vi "To String.vi"(6 "Encoding [No encoding]":refnum<class "CConfig Encoding.lvclass">, 7 "Persitant only?":bool, 8 "error in (no error)":errorcluster, 9 "Prev. Newline":string, 11 "Section Object in":refnum<class "CConfig Object.lvclass">) -> (0 "error out":errorcluster, 1 "Next Newline":string, 2 "String":string, 3 "Section Object out":refnum<class "CConfig Object.lvclass">)   [LabVIEW 2013, in "CConfig Object.lvclass"]
doc: "Copyright 2018, Carya Automatisering, Wiebe Walstra."
uses:
  CConfig Object.lvclass
  CConfig Encoding/CConfig Encoding.lvclass
  CConfig Object.lvclass/CConfig Object.ctl
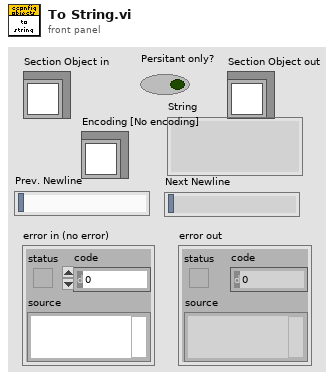
[diagram p1: front panel]
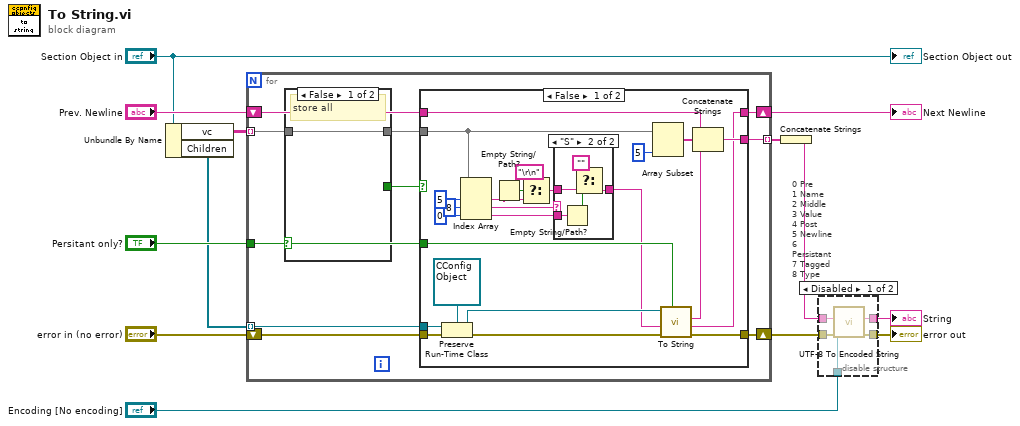
[diagram p0: block diagram]
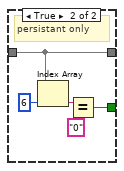
[diagram p3: hidden frame]
diagram:
  # "0 Pre\n1 Name\n2 Middle\n3 Value\n4 Post\n5 Newline\n6 Persistant\n7 Tagged\n8 Type"
  n1 = Unbundle By Name("Section Object in") -> ("vc"=w10:string[][], "Children"=w9:refnum<class>[])
  n2 = for {
    tunnel: [w23] -> w8 mode=indexing
    shift-right: [w22] -> w11
    shift-left: "error in (no error)" -> [w17]
    tunnel: "Persitant only?" -> [w15]
    tunnel: w10 -> [w19] mode=indexing
    tunnel: w9 -> [w18] mode=indexing
    shift-right: [w20] -> w4
    shift-left: "Prev. Newline" -> [w21]
    n3 = case shown="False" w15 {
      tunnel: w19 -> [w24 w25]
      tunnel: [_ w26] -> w16
      tunnel: [w24 w25] -> w14
      frame False {
        # "store all"
      }
      frame True {
        # "persistant only"
        n4 = Index Array(array=w25, index=6) -> (element=w27:string)
        n5 = Equal?(x=w27, y="0") -> (x = y?=w26:bool)
      }
    }
    n6 = case shown="False" w16 {
      tunnel: [w53 _] -> w23
      tunnel: w15 -> [w52 _]
      tunnel: [w51 w61] -> w22
      tunnel: w21 -> [w47 w60]
      tunnel: [w46 w60] -> w20
      tunnel: w14 -> [w40 _]
      tunnel: w17 -> [w45 w61]
      tunnel: w18 -> [w41 _]
      frame False {
        n7 = Preserve Run-Time Class(object in=w41, error in=w45, 2:refnum<class "CConfig Object.lvclass"> refnum ("Composite Object.lvclass")) -> (object out=w43:refnum<class "CConfig Object.lvclass">, error out=w44:errorcluster)
        n8 = Index Array(array=w40, index #1=5 ("index"), index #2=8 ("index"), index #3=0 ("index")) -> (element #1=w39:string, element #2=w33:string, element #3=w30:string)
        n9 = Empty String/Path?(string/path=w39) -> (empty?=w35:bool)
        n10 = Select(t="\r\n", s=w35, f=w39) -> (s? t:f=w32:string)
        n11 = case shown="\"S\"" w33 {
          tunnel: [w54 w56] -> w31
          tunnel: w32 -> [w54 w57]
          tunnel: w30 -> [_ w59]
          frame Default {
          }
          frame "S" {
            n12 = Empty String/Path?(string/path=w59) -> (empty?=w58:bool)
            n13 = Select(t="", s=w58, f=w57) -> (s? t:f=w56:string)
          }
        }
        n14 = Array Subset(array=w40, length=5 ("index")) -> (w49:string[])  [unwired: 1 in]
        n15 = call-dynamic "To String.vi"("Persitant only?"=w52, "error in (no error)"=w44, "Prev. Newline"=w31, "Section Object in"=w43) -> ("error out"=w51:errorcluster, "Next Newline"=w46:string, "String"=w50:string)  [unwired: 4 in, 1 out]
        n16 = Concatenate Strings(w47, w49, w50) -> (w53:string)
      }
      frame True {
      }
    }
  }
  "Next Newline" <- w4
  n17 = Concatenate Strings(w8) -> (w2:string)
  n18 = disable-structure shown="Disabled" {
    disable-tunnel: w11 -> [w66 w67]
    disable-tunnel: [w65 w67] -> w6
    disable-tunnel: [w64 w68] -> w3
    disable-tunnel: w2 -> [w63 w68]
    disable-tunnel: "Encoding [No encoding]" -> [w62 _]
    frame Disabled {
      n19 = call-dynamic "UTF-8 To Encoded String.vi"("error in (no error)"=w66, "UTF-8 string"=w63, "Encoding in"=w62) -> ("error out"=w65:errorcluster, "Encoded string"=w64:string)  [unwired: 6 in, 1 out]
    }
    frame Enabled {
    }
  }
  "error out" <- w6
  "String" <- w3
  "Section Object out" <- "Section Object in"
